vi "DB_Update.vi"   [LabVIEW 2020]
uses:
  <vilib>/addons/database/Connection.llb/DB Tools Open Connec (String).vi
  <vilib>/addons/database/NI_Database_API.lvlib
types:
  T1 = typedef "NI_Database_API.lvlib/Conn ObjectReference.ctl" = refnum<k1>
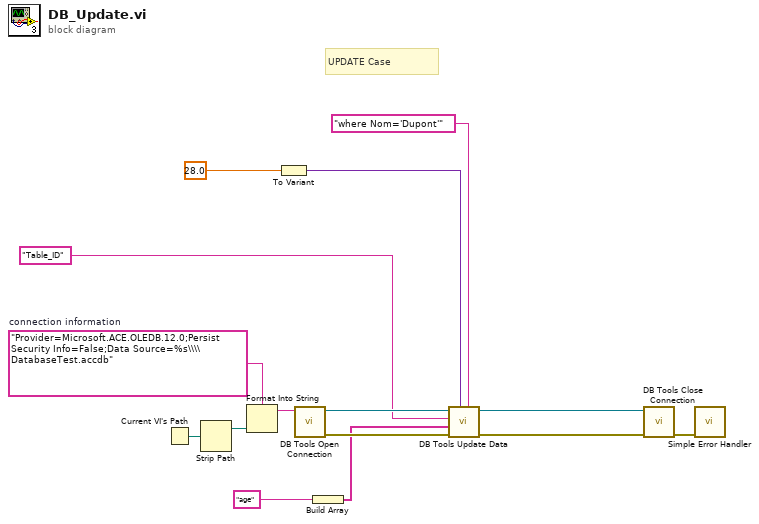
[diagram p0: block diagram]
diagram:
  w9 = "Provider=Microsoft.ACE.OLEDB.12.0;Persist Security Info=False;Data Source=%s\\\\DatabaseTest.accdb"  # connection information
  # "UPDATE Case"
  n1 = Current VI's Path() -> (path=w13:path)
  n2 = Strip Path(path=w13) -> (stripped path=w10:path)  [unwired: 1 out]
  n3 = Format Into String(format string=w9, w10) -> (resulting string=w11:string)  [unwired: 2 in, 1 out]
  n4 = To Variant(anything=sgl 28.0 ("age")) -> (Variant=w4:variant)
  n5 = call-poly <vilib>:"DB Tools Open Connection.vi"("connection information"=w11) -> ("error out"=w14:errorcluster, "connection reference"=w15:T1)  [unwired: 7 in]
  n6 = Build Array("age" ("String")) -> (w6:string[])
  n7 = call <vilib>:"DB Tools Update Data.vi"("condition"="where Nom='Dupont'" ("format string"), "data"=w4, "error in (no error)"=w14, "columns"=w6, "table"="Table_ID", "connection reference"=w15) -> ("error out"=w1:errorcluster, "connection reference out"=w2:T1)  [unwired: 4 in]
  n8 = call <vilib>:"DB Tools Close Connection.vi"("error in (no error)"=w1, "connection reference"=w2) -> ("error out"=w12:errorcluster)  [unwired: 5 in]
  n9 = call <vilib>:"Simple Error Handler.vi"("error in (no error)"=w12) -> ()  [unwired: 4 in, 5 out]
